vi "DrawContent.vi"(0 "In Image":T1, 1 "New Image":T1, 2 "Normalized Landmakers":u32[][](array[numeric]), 3 "VideoAccuracy [mm/px]":dbl format="%_6g") -> (7 "Distances":dbl[](array[numeric]), 8 "Out Image":T1)   [LabVIEW 2024]
uses:
  <vilib>/vision/Image Controls.llb/IMAQ Image.ctl
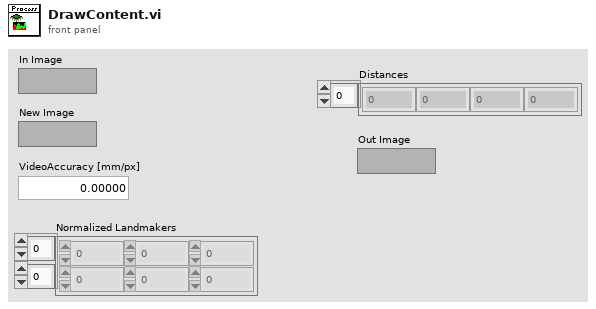
[diagram p1: front panel]
types:
  T1 = typedef "IMAQ Image.ctl" = refnum<image>
  T2 = typedef "#AntennaControlNumber.ctl" = enum16{"Ant1", "Ant2", "Ant3", "Ant4"}
  T3 = typedef "IMAQdx.ctl" = refnum<k21>
  T4 = cluster{"Reverse fingers":bool, "SelectingButton":bool, "Antenna":T2, "TestVsion":bool, "Camera source":T3, "AntDistance [mm]":dbl}
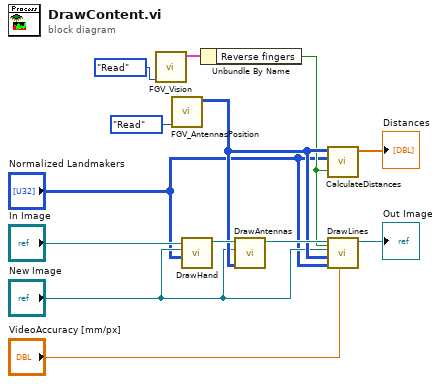
[diagram p0: block diagram]
diagram:
  n1 = call "FGV_Vision.vi"("Operation"=enum16{"Read", "Write"}."Read") -> ("OutVision"=w8:T4)  [unwired: 8 in]
  n2 = call "FGV_AntennasPosition.vi"("Type"=enum16{"Read", "Write"}."Read") -> ("AntennasPosition"=w10:u32[][])  [unwired: 10 in]
  n3 = call "DrawHand.vi"("Normalized Landmakers"="Normalized Landmakers", "New Image"="New Image", "In Image"="In Image") -> ("Out Image"=w13:T1)  [unwired: 8 in]
  n4 = Unbundle By Name(w8) -> ("Reverse fingers"=w7:bool)
  n5 = call "DrawAntennas.vi"("Coords"=w10, "New Image"="New Image", "In Image"=w13) -> ("Out Image"=w12:T1)  [unwired: 8 in]
  n6 = call "CalculateDistances.vi"("isReverse?"=w7, "Landmarkers Coordinates"="Normalized Landmakers", "Antenna Coordinates"=w10) -> ("Distances"=→"Distances":dbl[])  [unwired: 8 in]
  n7 = call "DrawLines.vi"("VideoAccuracy [mm/px]"="VideoAccuracy [mm/px]", "IsReverse?"=w7, "Landmarkers Coordinates"="Normalized Landmakers", "Antenna Coordinates"=w10, "New Image"="New Image", "In Image"=w12) -> ("Out Image"=→"Out Image":T1)  [unwired: 4 in]
